vi "setRootElement.vi"(8 "error in (no error)":errorcluster, 10 "RootElement":refnum<k20>, 11 "NativeXML in":refnum<class "NativeXML.lvclass">) -> (0 "error out":errorcluster, 3 "NativeXML out":refnum<class "NativeXML.lvclass">)   [LabVIEW 2011, in "Tools.lvlib" / "xml.lvlib" / "NativeXML.lvclass"]
uses:
  NativeXML.lvclass
  NativeXML.lvclass/NativeXML.ctl
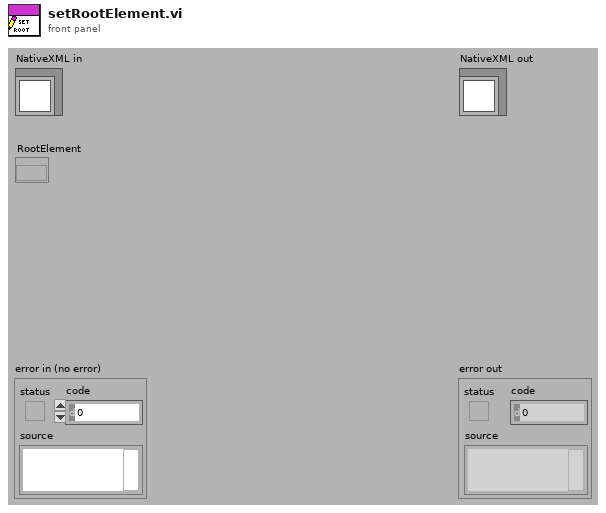
[diagram p1: front panel]
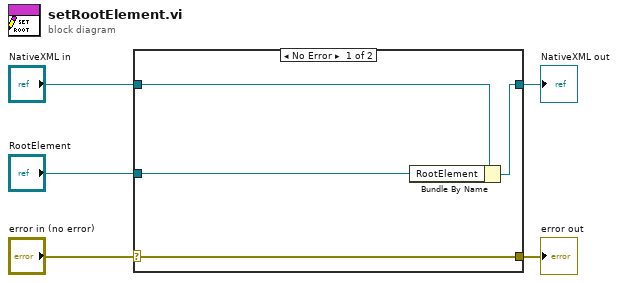
[diagram p0: block diagram]
diagram:
  n1 = case shown="No Error" "error in (no error)" {
    selector: "error in (no error)" -> [w9 w10]
    tunnel: [w9 w10] -> w4
    tunnel: [w7 w11] -> w2
    tunnel: "NativeXML in" -> [w8 w11]
    tunnel: "RootElement" -> [w6 _]
    frame No Error {
      n2 = Bundle By Name(cluster=w8, "RootElement"=w6) -> (w7:refnum<class "NativeXML.lvclass">)
    }
    frame Error {
    }
  }
  "error out" <- w4
  "NativeXML out" <- w2
